vi "XY Graph Save Graph Image.vi"(8 "Error In":errorcluster, 9 "Saved Image File Format":T1, 10 "Image File Path in":path, 11 "XYGraph in":refnum<vi>) -> (0 "Error Out":errorcluster, 2 "Image File Path out":path)   [LabVIEW 2021, in "XY Graph Add-Ons.lvlib"]
uses:
  XY Graph Add-Ons.lvlib
  Image/Image Save File Format.ctl
  Image/Selected Area in Object.ctl
  Image/Image.lvlib
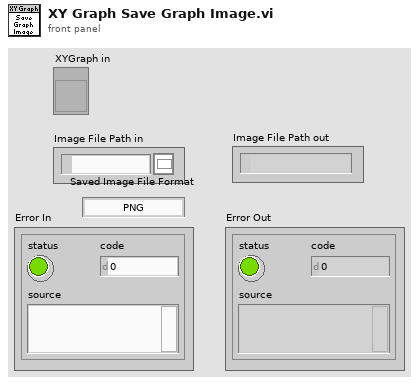
[diagram p1: front panel]
types:
  T1 = typedef "Image.lvlib/Image Save File Format.ctl" = enum16{"PNG", "JPEG", "BMP"}
  T2 = typedef "Image.lvlib/Selected Area in Object.ctl" = cluster{"Selected Area Position Left":i32, "Selected Area Position Top":i32, "Selected Area Size Height":u32, "Selected Area Size Width":u32, "Object Position Left":i32, "Object Position Top":i32}
  T3 = typedef "imagedata.ctl" = cluster{"image type":i32, "image depth":i32, "image":u8[], "mask":u8[], "colors":u32[], "Rectangle":cluster{"left":i16, "top":i16, "right":i16, "bottom":i16}}
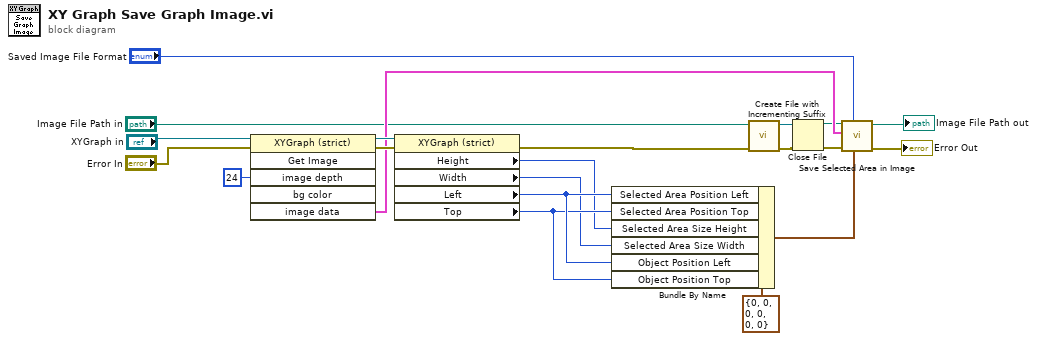
[diagram p0: block diagram]
diagram:
  n1 = invoke class="XYGraph (strict)" method="Get Image"(reference="XYGraph in", error in="Error In", "image depth"=24 ("Image Depth")) -> (reference out=w19:refnum<vi>, error out=w17:errorcluster, "image data"=w16:T3)  [unwired: 3 in, 3 out]
  n2 = property class="XYGraph (strict)"(reference=w19, error in=w17) -> (error out=w5:errorcluster, "Height"=w8:u32, "Width"=w7:u32, "Left"=w10:i32, "Top"=w9:i32)  [unwired: 1 out]
  n3 = Bundle By Name(cluster=T2 {"Selected Area Position Left"=0, "Selected Area Position Top"=0, "Selected Area Size Height"=0, "Selected Area Size Width"=0, "Object Position Left"=0, "Object Position Top"=0} ("Selected Area in Object"), "Selected Area Position Left"=w10, "Selected Area Position Top"=w9, "Selected Area Size Height"=w8, "Selected Area Size Width"=w7, "Object Position Left"=w10, "Object Position Top"=w9) -> (w11:T2)
  n4 = call <vilib>:"Create File with Incrementing Suffix.vi"("error in (no error)"=w5, "file path"="Image File Path in") -> ("error out"=w3:errorcluster, "refnum out"=w4:refnum<file>)  [unwired: 7 in, 1 out]
  n5 = Close File(refnum=w4, error in=w3) -> (path=w1:path, error out=w2:errorcluster)
  n6 = call "Save Selected Area in Image.vi"("Selected Area in Object"=w11, "Saved Image File Format"="Saved Image File Format", "error in (no error)"=w2, "Image Data"=w16, "File Path in"=w1) -> ("error out"=→"Error Out":errorcluster, "File Path out"=→"Image File Path out":path)  [unwired: 5 in]
